vi "EnqueueEconomyWash.vi"(11 "Queue in":refnum<queue>) -> (3 "queue out":refnum<queue>)   [LabVIEW 2018]
uses:
  MessageQueueData.ctl
  Command.ctl
  WashState.ctl
  Position.ctl
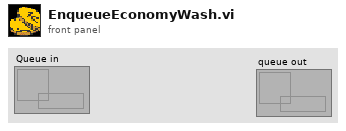
[diagram p1: front panel]
types:
  T1 = typedef "MessageQueueData.ctl" = cluster{"State":T2, "Data":variant}
  T2 = typedef "Command.ctl" = enum16{"Underbody Wash", "Soap Application", "Main High-Pressure Wash", "Clear Water Rinse", "Air Dry Cycle", "Stop"}
  T3 = typedef "WashState.ctl" = cluster{"Time Remaining":i32, "LastTickCount":i32, "Required Vehicle Position":T4}
  T4 = typedef "Position.ctl" = enum32{"Under Body Wash Position", "Main Wash Position", "Air Dry Position"}
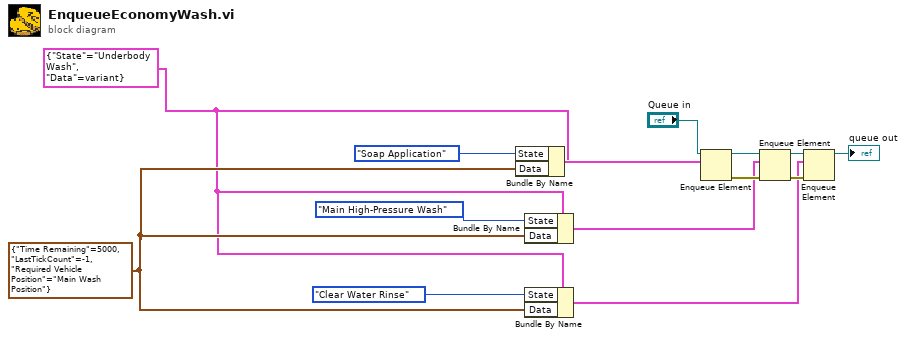
[diagram p0: block diagram]
diagram:
  w1 = T1 {"State"=enum."Underbody Wash", "Data"=variant}
  w2 = T3 {"Time Remaining"=5000, "LastTickCount"=-1, "Required Vehicle Position"=enum."Main Wash Position"} ("WashState")
  n1 = Bundle By Name(cluster=w1, "State"=Command."Soap Application" ("Command"), "Data"=w2) -> (w12:T1)
  n2 = Bundle By Name(cluster=w1, "State"=Command."Main High-Pressure Wash" ("Command"), "Data"=w2) -> (w3:T1)
  n3 = Bundle By Name(cluster=w1, "State"=Command."Clear Water Rinse" ("Command"), "Data"=w2) -> (w4:T1)
  n4 = Enqueue Element(queue="Queue in", element=w12) -> (queue out=w10:refnum<queue>, error out=w6:errorcluster)  [unwired: 2 in, 1 out]
  n5 = Enqueue Element(queue=w10, element=w3, error in (no error)=w6) -> (queue out=w9:refnum<queue>, error out=w5:errorcluster)  [unwired: 1 in, 1 out]
  n6 = Enqueue Element(queue=w9, element=w4, error in (no error)=w5) -> (queue out=→"queue out":refnum<queue>)  [unwired: 1 in, 2 out]
